vi "@destroy.vi"(8 "error in (no error)":errorcluster, 11 "dotnet_system_exec in":refnum<class "dotnet_system_exec.lvclass">) -> (0 "error out":errorcluster, 3 "dotnet_system_exec out":refnum<class "dotnet_system_exec.lvclass">)   [LabVIEW 2020, in "JKI dotNET System Exec.lvlib" / "dotnet_system_exec.lvclass"]
doc: "Stops the .NET System Process and destroy the necessary references.\n\n-----------------------------------------------\nJKI .NET System Exec 1.0.0.6\nJavier Ruiz - JKI\nCopyright (c) 2021, JKI\njki.net"
uses:
  dotnet_system_exec.lvclass
  dotnet_system_exec.lvclass/dotnet_system_exec.ctl
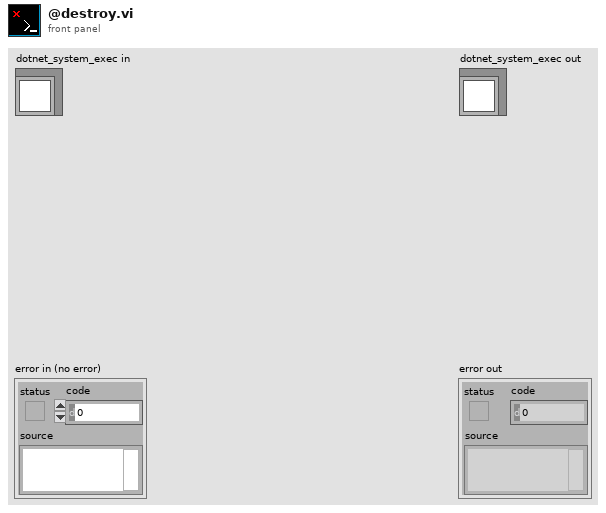
[diagram p1: front panel]
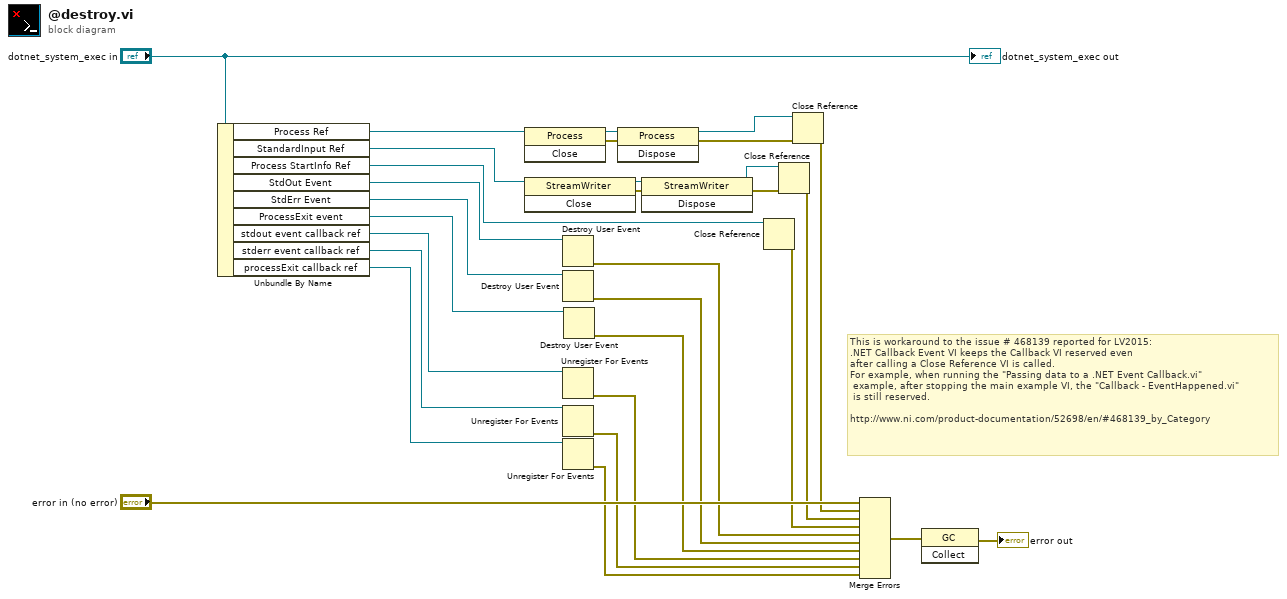
[diagram p0: block diagram]
diagram:
  # "This is workaround to the issue # 468139 reported for LV2015:\n.NET Callback Event VI keeps the Callback VI reserved even \nafter calling a Close Reference VI is called.\nFor example, when running the \"Passing data to a .NET Event Callback.vi\"\n example, after stopping the main example VI, the \"Callback - EventHappened.vi\"\n is still reserved.\n\nhttp://www.ni.com/product-documentation/52698/en/#468139_by_Category"
  n1 = Unbundle By Name("dotnet_system_exec in") -> ("Process Ref"=w8:refnum<k24>, "StandardInput Ref"=w19:refnum<k24>, "Process StartInfo Ref"=w18:refnum<k24>, "StdOut Event"=w16:refnum<user-event>, "StdErr Event"=w15:refnum<user-event>, "ProcessExit event"=w3:refnum<user-event>, "stdout event callback ref"=w12:refnum<k27>, "stderr event callback ref"=w11:refnum<k27>, "processExit callback ref"=w4:refnum<k27>)
  n2 = invoke class="Process" method="Close"(reference=w8) -> (reference out=w24:refnum<k24>, error out=w23:errorcluster)  [unwired: 2 in, 1 out]
  n3 = invoke class="StreamWriter" method="Close"(reference=w19) -> (reference out=w28:refnum<k24>, error out=w27:errorcluster)  [unwired: 2 in, 1 out]
  n4 = Destroy User Event(user event=w16) -> (error out=w14:errorcluster)  [unwired: 1 in]
  n5 = Destroy User Event(user event=w15) -> (error out=w13:errorcluster)  [unwired: 1 in]
  n6 = Unregister For Events(event registration refnum=w12) -> (error out=w10:errorcluster)  [unwired: 1 in]
  n7 = Unregister For Events(event registration refnum=w11) -> (error out=w9:errorcluster)  [unwired: 1 in]
  n8 = Unregister For Events(event registration refnum=w4) -> (error out=w1:errorcluster)  [unwired: 1 in]
  n9 = Destroy User Event(user event=w3) -> (error out=w2:errorcluster)  [unwired: 1 in]
  n10 = invoke class="Process" method="Dispose"(reference=w24, error in=w23) -> (reference out=w21:refnum<k24>, error out=w22:errorcluster)  [unwired: 1 in, 1 out]
  n11 = invoke class="StreamWriter" method="Dispose"(reference=w28, error in=w27) -> (reference out=w25:refnum<k24>, error out=w26:errorcluster)  [unwired: 1 in, 1 out]
  n12 = Close Reference(reference=w18) -> (error out=w17:errorcluster)  [unwired: 1 in]
  n13 = Close Reference(reference=w25, error in (no error)=w26) -> (error out=w20:errorcluster)
  n14 = Close Reference(reference=w21, error in (no error)=w22) -> (error out=w7:errorcluster)
  n15 = Merge Errors("error in (no error)", w7, w20, w17, w14, w13, w2, w10, w9, w1) -> (w6:errorcluster)
  n16 = invoke class="GC" method="Collect"(error in=w6) -> (error out=→"error out":errorcluster)  [unwired: 2 in, 2 out]
  "dotnet_system_exec out" <- "dotnet_system_exec in"
